vi "State Tracker for Debug.vi"(11 "State":string) -> ()   [LabVIEW 2012]
uses:
  <vilib>/Rock Robotics/WPI/DriverStation/DriverStationLCD/WPI_DriverStationLCDLCDLine.ctl
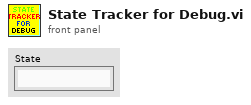
[diagram p1: front panel]
types:
  T1 = typedef "WPI_DriverStationLCDLCDLine.ctl" = enum16{"Main - Line 1", "User - Line 2", "User - Line 3", "User - Line 4", "User - Line 5", "User - Line 6"}
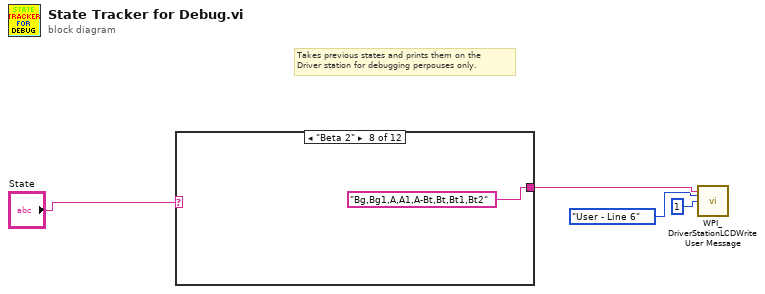
[diagram p0: block diagram]
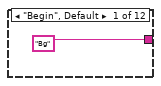
[diagram p2: hidden frame]
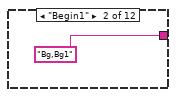
[diagram p3: hidden frame]
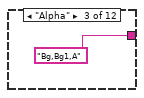
[diagram p4: hidden frame]
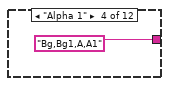
[diagram p5: hidden frame]
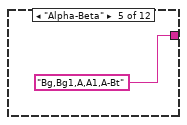
[diagram p6: hidden frame]
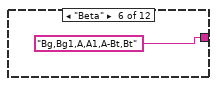
[diagram p7: hidden frame]
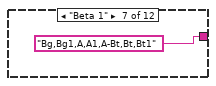
[diagram p8: hidden frame]
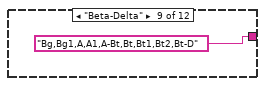
[diagram p9: hidden frame]
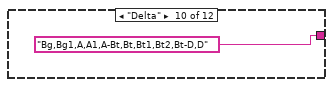
[diagram p10: hidden frame]
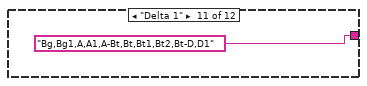
[diagram p11: hidden frame]
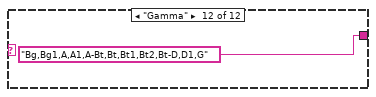
[diagram p12: hidden frame]
diagram:
  # "Takes previous states and prints them on the\nDriver station for debugging perpouses only."
  n1 = case shown="\"Beta 2\"" "State" {
    tunnel: ["Bg" "Bg,Bg1" "Bg,Bg1,A" "Bg,Bg1,A,A1" "Bg,Bg1,A,A1,A-Bt" "Bg,Bg1,A,A1,A-Bt,Bt" "Bg,Bg1,A,A1,A-Bt,Bt,Bt1" "Bg,Bg1,A,A1,A-Bt,Bt,Bt1,Bt2" "Bg,Bg1,A,A1,A-Bt,Bt,Bt1,Bt2,Bt-D" "Bg,Bg1,A,A1,A-Bt,Bt,Bt1,Bt2,Bt-D,D" "Bg,Bg1,A,A1,A-Bt,Bt,Bt1,Bt2,Bt-D,D1" "Bg,Bg1,A,A1,A-Bt,Bt,Bt1,Bt2,Bt-D,D1,G"] -> w4
    frame "Begin", Default {
    }
    frame "Begin1" {
    }
    frame "Alpha" {
    }
    frame "Alpha 1" {
    }
    frame "Alpha-Beta" {
    }
    frame "Beta" {
    }
    frame "Beta 1" {
    }
    frame "Beta 2" {
    }
    frame "Beta-Delta" {
    }
    frame "Delta" {
    }
    frame "Delta 1" {
    }
    frame "Gamma" {
    }
  }
  n2 = call <vilib>:"WPI_DriverStationLCDWrite User Message.vi"("line text"=w4, "line"=WPI_DriverStationLCDLCDLine."User - Line 6", "starting column"=i8 1) -> ()  [unwired: 12 in, 1 out]
